vi "Temperatue Controller SelfTest.vi"(8 "error in":errorcluster) -> (0 "error out":errorcluster, 2 "Report Text":string, 3 "OK":bool)   [LabVIEW 2023, in "LTT_TeststandSteptypes.lvlib"]
uses:
  LTT_TeststandSteptypes.lvlib
  HardwareAbstractionLayer_LVOOP/Modbus/Modbus_class/Modbus.lvclass
  179f56aa-43f5-41aa-8ac2-b289e563d779.vi
  HardwareAbstractionLayer_LVOOP/Database/Database.lvclass
  HardwareAbstractionLayer_LVOOP/Database/SQL Public VI/Control/DB Options.ctl
  <userlib>/_OpenG.lib/error/error.llb/openg_error.lvlib
panel:
  out "Data":i16[](array[numeric])
  out "Array":i32[](array[numeric])
  in  "Modbus RTU":T1={"unit ID"=1, "serial type"=enum."RTU", "baud rate"=9600, "parity (even)"=2, "flow control (none)"=0, "VISA resource name"=""} {"flow control (none)" items=["None", "XON/XOFF", "RTS/CTS", "XON/XOFF & RTS/CTS", "DTR/DSR", "XON/XOFF & DTR/DSR"]; "parity (even)" items=["None", "Odd", "Even", "Mark", "Space"]}
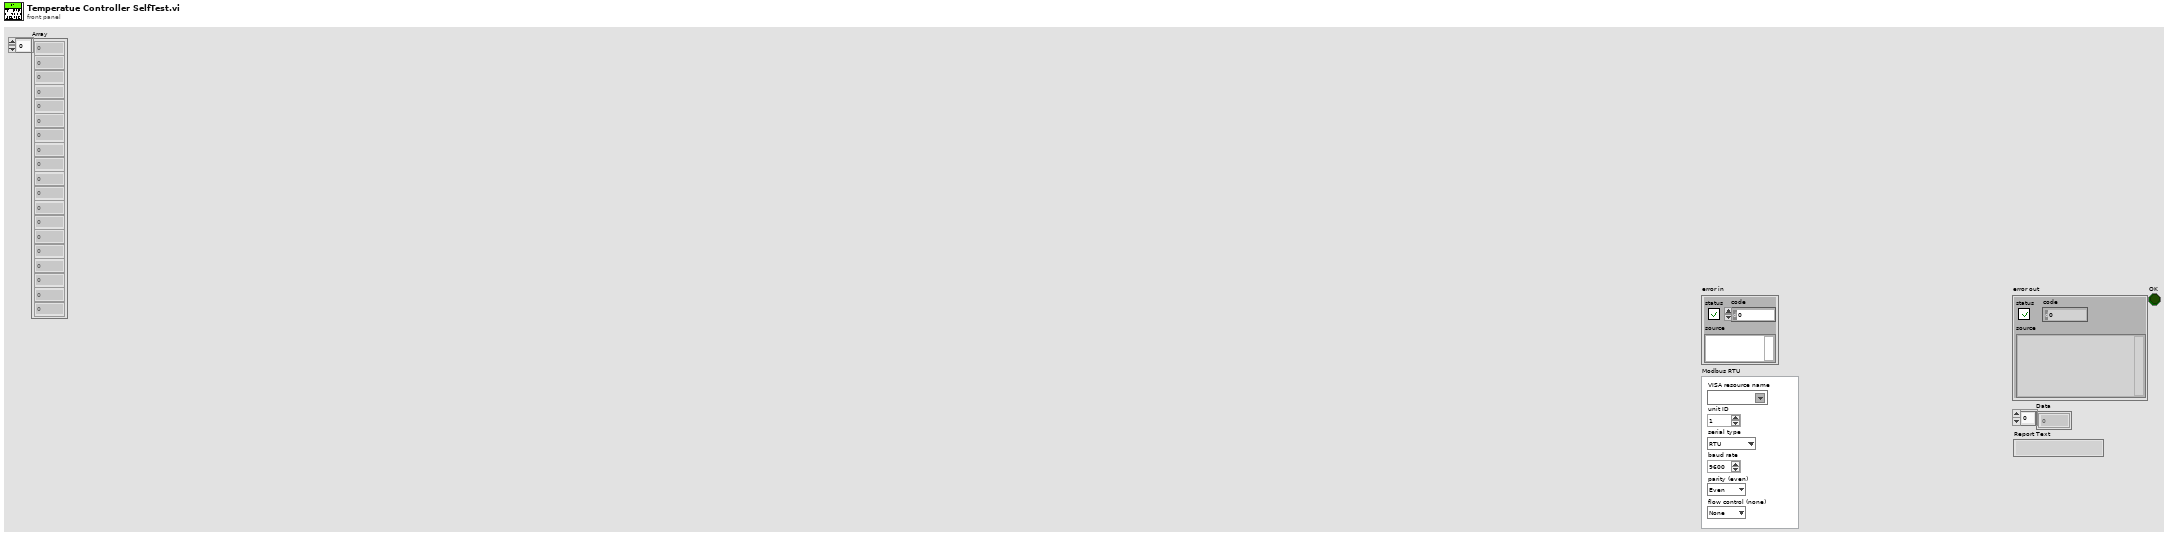
[diagram p1: front panel]
types:
  T1 = cluster{"unit ID":u8, "serial type":enum16{"RTU", "ASCII"}, "baud rate":u32, "parity (even)":u16, "flow control (none)":u16, "VISA resource name":refnum<visa-resource-name>}
  T2 = typedef "HardwareAbstractionLayer_LVOOP.lvlib/Database.lvclass/DB Options.ctl" = enum16{"Init", "Select Data", "Insert Data", "Update Data", "Delete Data", "Execute Query", "Create Schema", "Create Table", "List Tables", "List Columns", "Close"}
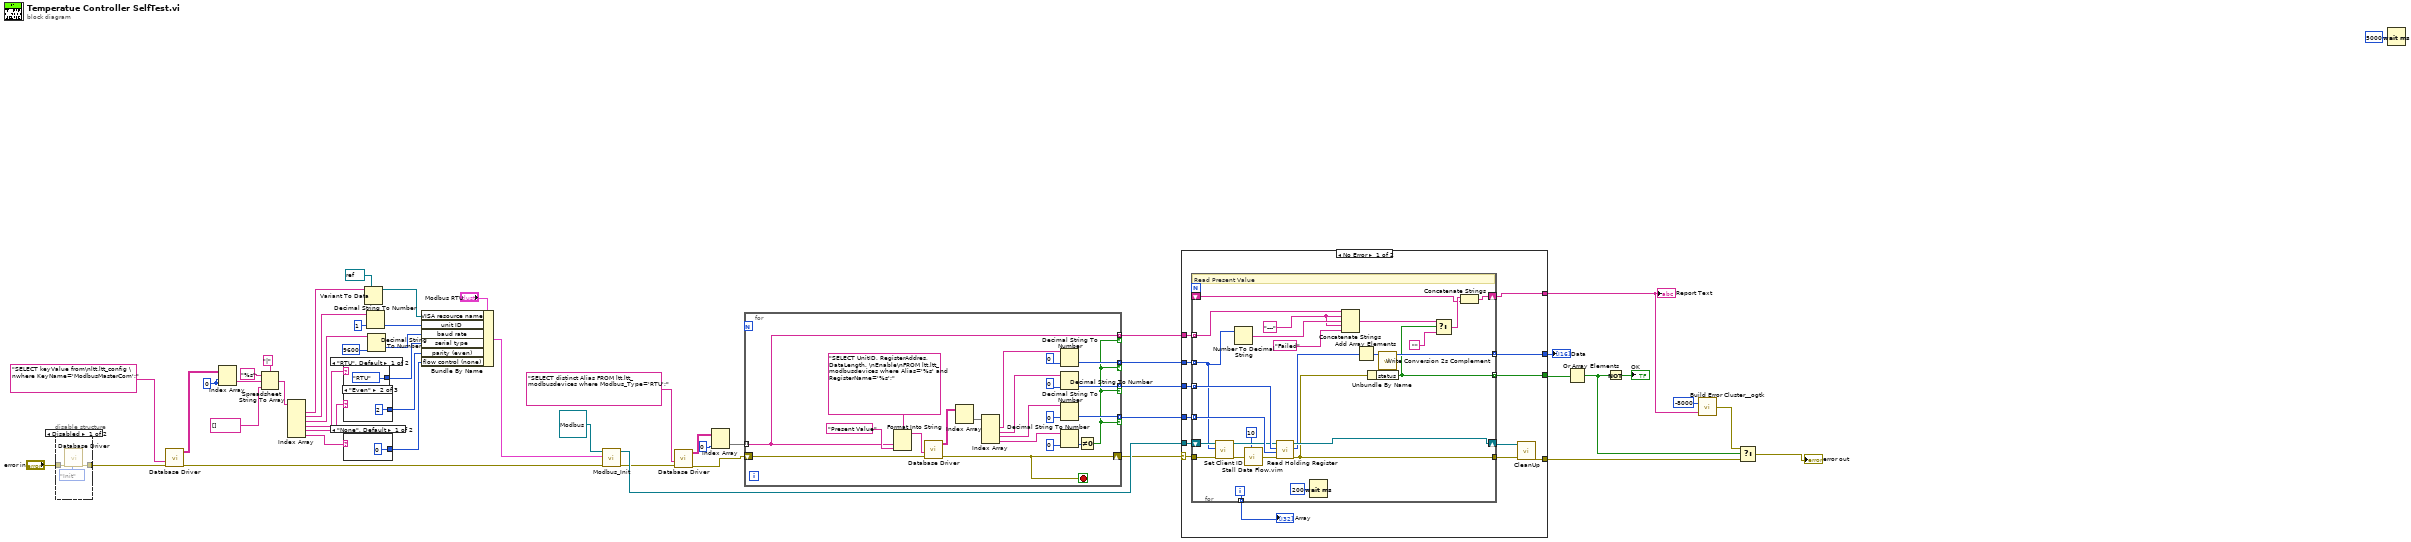
[diagram p0: block diagram]
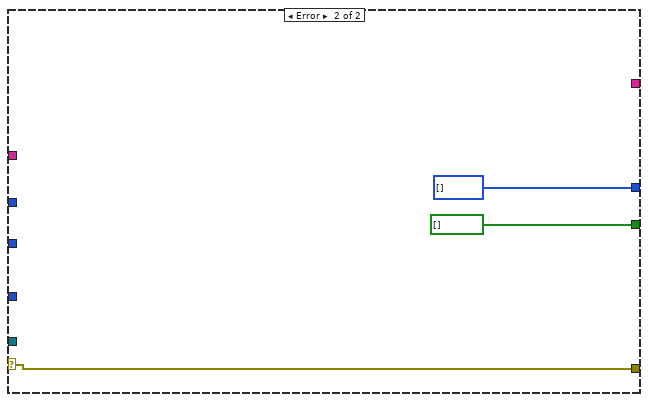
[diagram p2: hidden frame]
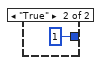
[diagram p4: hidden frame]
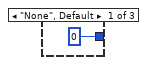
[diagram p5: hidden frame]
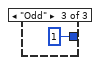
[diagram p6: hidden frame]
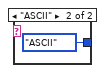
[diagram p7: hidden frame]
diagram:
  w48 = 0 ("index (row)")
  n1 = disable-structure shown="Disabled" {
    disable-tunnel: "error in" -> [w54 w55]
    disable-tunnel: [w53 w55] -> w17
    frame Disabled {
      n2 = call "Database Driver.vi"("Options"=DB_Options."Init", "error in"=w54) -> ("error out"=w53:errorcluster)  [unwired: 6 in, 3 out]
    }
    frame Enabled {
    }
  }
  n3 = call "Database Driver.vi"("error in"=w17, "SQL query"="SELECT keyValue from\nltt.ltt_config \nwhere KeyName='ModbusMasterCom';") -> ("error out"=w14:errorcluster, "data"=w49:string[][])  [unwired: 6 in, 2 out]
  n4 = Index Array(array=w49, index (row)=w48, index (col)=w48) -> (element=w47:string)
  n5 = Spreadsheet String To Array(delimiter (Tab)="|" ("format string"), format string="%s", spreadsheet string=w47, array type (2D Dbl)=string[] []) -> (array=w45:string[])
  n6 = Index Array(array=w45) -> (element #1=w30:string, element #2=w43:string, element #3=w40:string, element #4=w37:string, element #5=w35:string, element #6=w34:string)  [unwired: 6 in]
  n7 = case shown="\"Even\"" w35 {
    tunnel: [u16 0 ("parity (even)") u16 2 ("parity (even)") u16 1 ("parity (even)")] -> w33
    frame "None", Default {
    }
    frame "Even" {
    }
    frame "Odd" {
    }
  }
  n8 = case shown="\"None\", Default" w34 {
    tunnel: [u16 0 ("flow control (none)") u16 1 ("flow control (none)")] -> w32
    frame "None", Default {
    }
    frame "True" {
    }
  }
  n9 = case shown="\"RTU\", Default" w37 {
    tunnel: [enum16{"RTU", "ASCII"}."RTU" ("serial type") enum16{"RTU", "ASCII"}."ASCII" ("serial type")] -> w36
    frame "RTU", Default {
    }
    frame "ASCII" {
    }
  }
  n10 = Variant To Data(type=refnum<visa-resource-name> refnum ("VISA resource name"), Variant=w30) -> (data=w29:refnum<visa-resource-name>)  [unwired: 1 in, 1 out]
  n11 = Decimal String To Number(string=w43, default (0L)=u8 1 ("unit ID")) -> (number=w41:u8)  [unwired: 1 in, 1 out]
  n12 = Decimal String To Number(string=w40, default (0L)=u32 9600 ("baud rate")) -> (number=w39:u32)  [unwired: 1 in, 1 out]
  n13 = Bundle By Name(cluster="Modbus RTU", "VISA resource name"=w29, "unit ID"=w41, "baud rate"=w39, "serial type"=w36, "parity (even)"=w33, "flow control (none)"=w32) -> (w15:T1)
  n14 = call "Modbus_Init.vi"("error in (no error)"=w14, "Modbus RTU"=w15, "object in"=refnum<class "Modbus.lvclass"> refnum ("VT_LTT.lvlib:Modbus")) -> ("error out"=w22:errorcluster, "object out"=w25:refnum<class "Modbus.lvclass">)  [unwired: 7 in]
  n15 = call "Database Driver.vi"("error in"=w22, "SQL query"="SELECT distinct Alias FROM ltt.ltt_modbusdevices where Modbus_Type='RTU';") -> ("error out"=w11:errorcluster, "data"=w23:string[][])  [unwired: 6 in, 2 out]
  n16 = Index Array(array=w23, index (col)=0 ("disabled index (col)")) -> (element=w12:string[])  [unwired: 1 in]
  n17 = for {
    tunnel: w12 -> [w64] mode=indexing
    tunnel: [w72] -> w20 mode=indexing if=w63
    tunnel: [w71] -> w19 mode=indexing if=w63
    tunnel: [w70] -> w18 mode=indexing if=w63
    shift-right: [w69] -> w21
    shift-left: w11 -> [w68]
    tunnel: [w64] -> w13 mode=indexing if=w63
    stop <- w69 stop-if-true
    n18 = Format Into String(format string="SELECT UnitID, RegisterAddres, DataLength, \nEnable\nFROM ltt.ltt_modbusdevices where Alias='%s' and RegisterName='%s';", w64, "Present Value" ("input 2")) -> (resulting string=w83:string)  [unwired: 2 in, 1 out]
    n19 = call "Database Driver.vi"("error in"=w68, "SQL query"=w83) -> ("error out"=w69:errorcluster, "data"=w82:string[][])  [unwired: 6 in, 2 out]
    n20 = Index Array(array=w82) -> (element=w81:string[])  [unwired: 2 in]
    n21 = Index Array(array=w81) -> (element #1=w80:string, element #2=w77:string, element #3=w76:string, element #4=w66:string)  [unwired: 4 in]
    n22 = Decimal String To Number(string=w80, default (0L)=u8 0 ("Slave unit ID")) -> (number=w72:u8)  [unwired: 1 in, 1 out]
    n23 = Decimal String To Number(string=w77, default (0L)=u16 0 ("starting address")) -> (number=w71:u16)  [unwired: 1 in, 1 out]
    n24 = Decimal String To Number(string=w76, default (0L)=u16 0 ("number of inputs")) -> (number=w70:u16)  [unwired: 1 in, 1 out]
    n25 = Decimal String To Number(string=w66, default (0L)=u16 0 ("number of inputs")) -> (number=w65:u16)  [unwired: 1 in, 1 out]
    n26 = Not Equal To 0?(x=w65) -> (x != 0?=w63:bool)
  }
  n27 = case shown="No Error" w21 {
    selector: w21 -> [w96 w125]
    tunnel: w25 -> [w95 _]
    tunnel: w20 -> [w94 _]
    tunnel: w19 -> [w93 _]
    tunnel: w18 -> [w92 _]
    tunnel: w13 -> [w90 _]
    tunnel: [w87 w125] -> w3
    tunnel: [w86 bool[] []] -> w8
    tunnel: [w85 i16[] []] -> w9
    tunnel: [w84 _] -> w5
    frame No Error {
      n28 = for {
        tunnel: w94 -> [w104] mode=indexing
        shift-right: [w120] -> w88
        shift-left: w95 -> [w121]
        tunnel: w93 -> [w118] mode=indexing
        tunnel: w92 -> [w117] mode=indexing
        tunnel: [w116] -> w91 mode=indexing
        tunnel: w90 -> [w105] mode=indexing
        tunnel: [w108] -> w85 mode=indexing
        tunnel: [w107] -> w86 mode=indexing
        shift-right: [w98] -> w84
        shift-left: _ -> [w97]
        tunnel: w96 -> [w122]
        tunnel: [w109] -> w89
        i -> [w116]
        w100 = "---" ("string")
        # "Read Present Value"
        n29 = call-dynamic "Set Client ID.vi"("error in (no error)"=w122, "Slave unit ID"=w104, "Modbus in"=w121) -> ("error out"=w115:errorcluster, "Modbus out"=w114:refnum<class "Modbus.lvclass">)  [unwired: 7 in]
        n30 = Number To Decimal String(number=w104) -> (decimal integer string=w103:string)  [unwired: 1 in]
        n31 = call "Stall Data Flow.vim"("value in"=w115, "milliseconds to wait"=u32 10) -> ("value out"=w113:errorcluster)  [unwired: 1 out]
        n32 = call-dynamic "Read Holding Register.vi"("error in (no error)"=w113, "number of inputs"=w117, "starting address"=w118, "Modbus in"=w114) -> ("error out"=w109:errorcluster, "register values"=w110:u16[], "Modbus out"=w120:refnum<class "Modbus.lvclass">)  [unwired: 5 in]
        n33 = Wait (ms)(milliseconds to wait=u32 200) -> ()  [unwired: 1 out]
        n34 = Concatenate Strings(w105, w100, w103, w100, "Failed" ("string")) -> (w102:string)
        n35 = Add Array Elements(numeric array=w110) -> (sum=w111:u16)
        n36 = Unbundle By Name(w109) -> ("status"=w107:bool)
        n37 = call "Write Conversion 2s Complement.vi"("Set Data Input"=w111) -> ("Coversion Data Output"=w108:i16)  [unwired: 10 in]
        n38 = Select(t=w102, s=w107, f="") -> (s? t:f=w101:string)
        n39 = Concatenate Strings(w101, w97) -> (w98:string)
      }
      "Array" <- w91
      n40 = call-dynamic "CleanUp.vi"("object in"=w88, "error in (no error)"=w89) -> ("error out"=w87:errorcluster)  [unwired: 16 in, 1 out]
    }
    frame Error {
    }
  }
  "Data" <- w9
  "Report Text" <- w5
  n41 = Or Array Elements(Boolean array=w8) -> (logical OR=w4:bool)
  n42 = Not(x=w4) -> (.not. x?=→"OK":bool)
  n43 = call <userlib>:"Build Error Cluster__ogtk.vi"("String to Prepend to source (\"\")"=w5, "code"=-8000) -> ("error out"=w7:errorcluster)
  n44 = Select(t=w7, s=w4, f=w3) -> (s? t:f=→"error out":errorcluster)
  n45 = Wait (ms)(milliseconds to wait=u32 5000) -> ()  [unwired: 1 out]
